vi "LVDimInterface.dic_command_service.vi"(1 "commandName":string, 3 "data":string, 5 "error in (no error)":errorcluster, 7 "safeMode":bool=TRUE) -> (15 "success":i32, 19 "error out":errorcluster)   [LabVIEW 2013, in "LVDimInterface.lvlib"]
doc: "This routine requests the execution of a command by a server, address and size contain the command parameters. This implies contacting the name server (if the command in not know already) and then contacting directly the server. This routine does not report back the completion of the command since these operations are only scheduled and may complete asynchronously. \nIf the server is not responding the command is discarded (in order to avoid having it sent later when it might not be desired anymore). \n\nThis routine allows clients (user interfaces for ex.) to send commands to be executed by the servers.\n\nHistory: 16-DEC-2005, Dietrich Beck\n\nCopyright (C)\nGesellschaft für Schwerionenforschung, GSI\nPlanckstr. 1\n64291 Darmstadt\nGermany\n\nContact: D.Beck@gsi.de \n\nThis program is free software; you can redistribute it and/or modify it under the terms of the \nGNU General Public License as published by the Free Software Foundation; either version 2 of the license, or (at your option) any later version.\n\nThis program is distributed in the hope that it will be useful, but WITHOUT ANY WARRANTY; without even the implied warranty of MERCHANTABILITY or FITNESS FOR A PARTICULAR PURPOSE. See the GNU General License for more details (http://www.gnu.org).\n\nGesellschaft für Schwerionenforschung, GSI\nPlanckstr. 1, 64291 Darmstadt, Germany\nFor all questions and ideas contact D. Beck.\nLast update: 16-DEC-2005"
uses:
  LVDimInterface.lvlib
  bin/libDimWrapper.dll
  C/GPL/Projects/DimLVEvent/bin/libDimWrapper.so
  C/GPL/Projects/DimLVEvent/bin/libDimWrapperSPL.dll
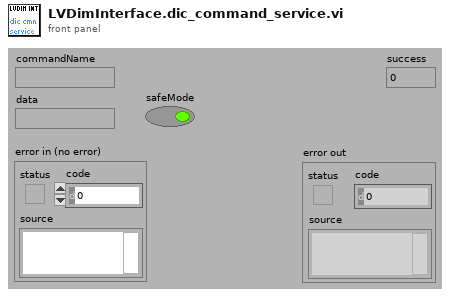
[diagram p1: front panel]
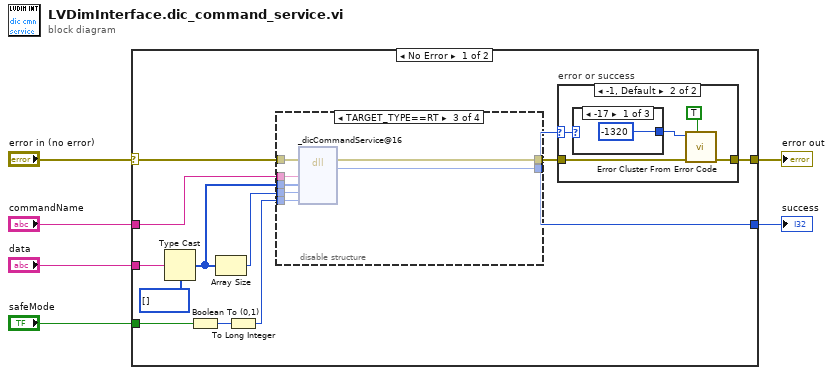
[diagram p0: block diagram]
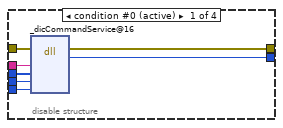
[diagram p2: hidden frame]
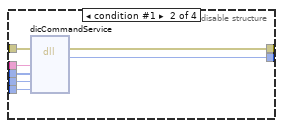
[diagram p3: hidden frame]
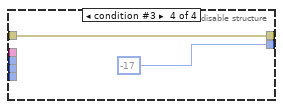
[diagram p4: hidden frame]
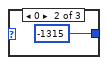
[diagram p6: hidden frame]
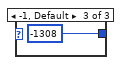
[diagram p7: hidden frame]
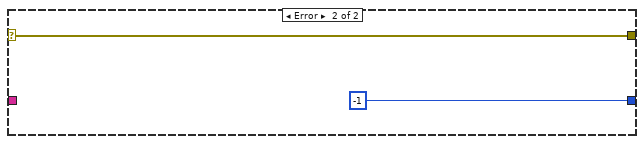
[diagram p8: hidden frame]
diagram:
  n1 = case shown="No Error" "error in (no error)" {
    selector: "error in (no error)" -> [w8 w51]
    tunnel: "commandName" -> [w18 _]
    tunnel: "data" -> [w13 _]
    tunnel: [w15 -1 ("success")] -> w4
    tunnel: [w16 w51] -> w3
    tunnel: "safeMode" -> [w11 _]
    frame No Error {
      n2 = Type Cast(type=i8[] [], x=w13) -> (*(type *) &x=w12:i8[])
      n3 = Boolean To (0,1)(Boolean=w11) -> (0, 1=w10:i16)
      n4 = Array Size(array=w12) -> (size(s)=w17:i32)
      n5 = To Long Integer(number=w10) -> (32bit integer=w9:i32)
      n6 = disable-structure "Conditional Disable Structure" shown="TARGET_TYPE==RT" {
        disable-tunnel: w18 -> [w25 w32 w39 _]
        disable-tunnel: w17 -> [w24 w31 w38 _]
        disable-tunnel: [w23 w30 w37 -17 ("success")] -> w15
        disable-tunnel: w12 -> [w22 w29 w36 _]
        disable-tunnel: w9 -> [w21 w28 w35 _]
        disable-tunnel: w8 -> [w20 w27 w34 w40]
        disable-tunnel: [w19 w26 w33 w40] -> w7
        frame condition #0 (active) {
          n7 = dll-call lib="C:/User/Brand/LVP/Submodules/DimLVEvent/bin/libDimWrapper.dll" fn="_dicCommandService@16"(error in=w20, "name"=w25, "data"=w22, "size"=w24, "safeMode"=w21) -> (error out=w19:errorcluster, "success"=w23:i32)  [unwired: 6 in, 1 out]
        }
        frame condition #1 {
          n8 = dll-call lib="F:/LVSCC/C/GPL/Projects/DimLVEvent/bin/libDimWrapper.so" fn="dicCommandService" label="libDimWrapper.dll:_dicCommandService@16"(error in=w27, "name"=w32, "data"=w29, "size"=w31, "safeMode"=w28) -> (error out=w26:errorcluster, "success"=w30:i32)  [unwired: 6 in, 1 out]
        }
        frame condition #2 {
          n9 = dll-call lib="C:/User/Brand/SVN/C/GPL/Projects/DimLVEvent/bin/libDimWrapperSPL.dll" fn="_dicCommandService@16"(error in=w34, "name"=w39, "data"=w36, "size"=w38, "safeMode"=w35) -> (error out=w33:errorcluster, "success"=w37:i32)  [unwired: 6 in, 1 out]
        }
        frame condition #3 {
        }
      }
      n10 = case "error or success" shown="-1, Default" w15 {
        selector: w15 -> [_ w47]
        tunnel: w7 -> [w42 w45]
        tunnel: [w42 w46] -> w16
        frame 1 {
        }
        frame -1, Default {
          n11 = case shown="-17" w47 {
            tunnel: [-1320 ("code") -1315 ("code") -1308 ("code")] -> w44
            frame -17 {
            }
            frame 0 {
            }
            frame -1, Default {
            }
          }
          n12 = call <vilib>:"Error Cluster From Error Code.vi"("show call chain? (False)"=TRUE ("status"), "error in (no error)"=w45, "error code (0)"=w44) -> ("error out"=w46:errorcluster)  [unwired: 6 in]
        }
      }
    }
    frame Error {
    }
  }
  "success" <- w4
  "error out" <- w3
